vi "RobotSimulator.vi"() -> ()   [LabVIEW 2020]
uses:
  <vilib>/Utility/inputDevices.llb/joystickAcquire.vi
  <vilib>/Utility/inputDevices.llb/closeJoystick.vi
panel:
  out "?":dbl(knob) scale=-10.0..10.0
  out "Velocidade":dbl
  out "Trás Esq.":bool
  out "Frente Dir.":bool
  out "Trás Dir.":bool
  out "Frente Esq.":bool
  out "joystick info":T1(array[cluster])
  out "direction info":T2
  out "button info":T3
  out "axis info":T4
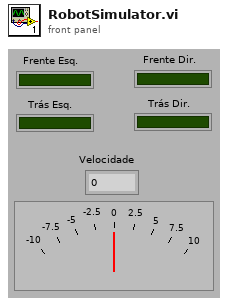
[diagram p1: front panel]
types:
  T1 = cluster{"axes total":u32, "buttons total":u32, "pov total":u32, "device name":string}[]
  T2 = cluster{"pov 1":i32, "pov 2":i32, "pov 3":i32, "pov 4":i32}
  T3 = cluster{"button 1":bool, "button 2":bool, "button 3":bool, "button 4":bool, "button 5":bool, "button 6":bool, "button 7":bool, "button 8":bool, "button 9":bool, "button 10":bool, "button 11":bool, "button 12":bool, "button 13":bool, "button 14":bool, "button 15":bool, "button 16":bool, "button 17":bool, "button 18":bool, "button 19":bool, "button 20":bool, "button 21":bool, "button 22":bool, "button 23":bool, "button 24":bool, "button 25":bool, "button 26":bool, "button 27":bool, "button 28":bool, "button 29":bool, "button 30":bool, "button 31":bool, "button 32":bool}
  T4 = cluster{"X axis":i32, "Y axis":i32, "Z axis":i32, "X axis rotation":i32, "Y axis rotation":i32, "Z axis rotation":i32, "U axis":i32, "V axis":i32}
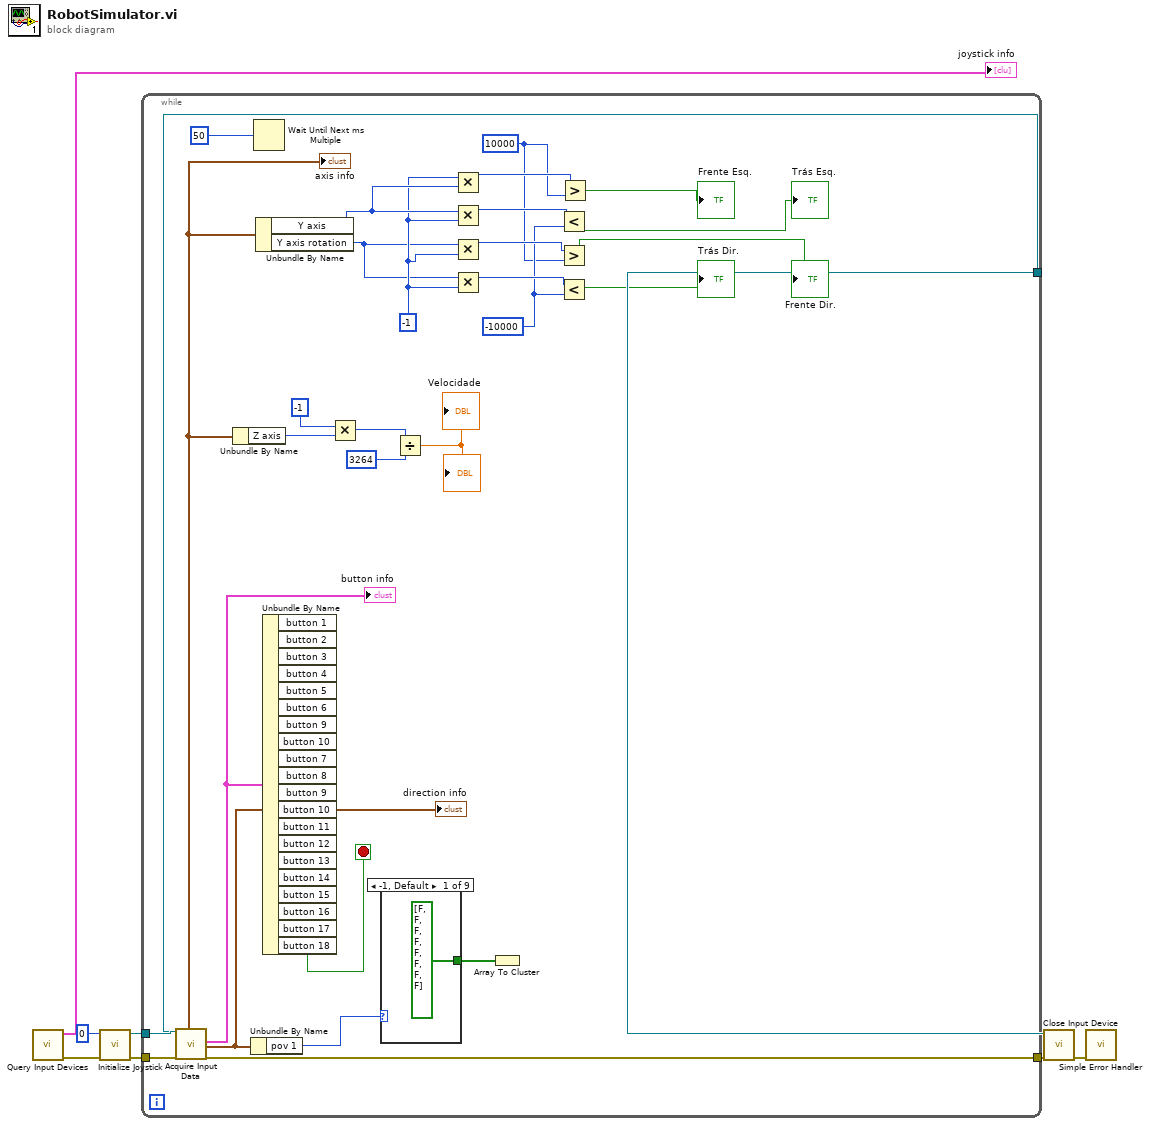
[diagram p0: block diagram]
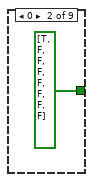
[diagram p2: hidden frame]
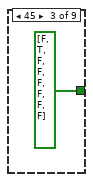
[diagram p3: hidden frame]
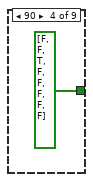
[diagram p4: hidden frame]
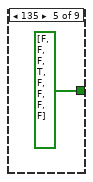
[diagram p5: hidden frame]
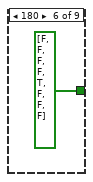
[diagram p6: hidden frame]
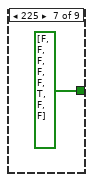
[diagram p7: hidden frame]
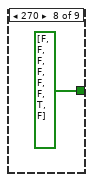
[diagram p8: hidden frame]
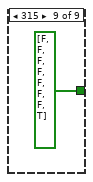
[diagram p9: hidden frame]
diagram:
  n1 = call <vilib>:"Query Input Devices.vi"() -> ("error out"=w2:errorcluster, "joystick info"=→"joystick info":T1)  [unwired: 1 in, 9 out]
  n2 = call <vilib>:"Initialize Joystick.vi"("error in (no error)"=w2, "device index"=0) -> ("error out"=w6:errorcluster, "device ID"=w7:refnum<k1>)  [unwired: 8 out]
  n3 = while {
    tunnel: w7 -> [w37]
    tunnel: w6 -> [w36]
    tunnel: [w35] -> w5
    tunnel: [w30] -> w4
    stop <- w29 stop-if-true
    w15 = 10000
    w16 = -10000
    w25 = -1
    n4 = call-poly <vilib>:"Acquire Input Data.vi"("device ID"=w37, "error in (no error)"=w36) -> ("device ID"=w35:refnum<k1>, "axis info"=w27:T4, "button info"=w34:T3, "direction info"=w33:T2, "error out"=w30:errorcluster)  [unwired: 13 out]
    "axis info" <- w27
    "button info" <- w34
    "direction info" <- w33
    n5 = Unbundle By Name(w27) -> ("Z axis"=w12:i32)
    n6 = Unbundle By Name(w33) -> ("pov 1"=w32:i32)
    n7 = Wait Until Next ms Multiple(millisecond multiple=u32 50) -> ()  [unwired: 1 out]
    n8 = Unbundle By Name(w27) -> ("Y axis"=w26:i32, "Y axis rotation"=w24:i32)
    n9 = Unbundle By Name(w34) -> ("button 7"=w29:bool)  [unwired: 19 out]
    n10 = Multiply(x=w12, y=-1) -> (x*y=w11:i32)
    n11 = case shown="-1, Default" w32 {
      tunnel: [bool[] [FALSE, FALSE, FALSE, FALSE, FALSE, FALSE, FALSE, FALSE] ("Array") bool[] [TRUE, FALSE, FALSE, FALSE, FALSE, FALSE, FALSE, FALSE] ("Array") bool[] [FALSE, TRUE, FALSE, FALSE, FALSE, FALSE, FALSE, FALSE] ("Array") bool[] [FALSE, FALSE, TRUE, FALSE, FALSE, FALSE, FALSE, FALSE] ("Array") bool[] [FALSE, FALSE, FALSE, TRUE, FALSE, FALSE, FALSE, FALSE] ("Array") bool[] [FALSE, FALSE, FALSE, FALSE, TRUE, FALSE, FALSE, FALSE] ("Array") bool[] [FALSE, FALSE, FALSE, FALSE, FALSE, TRUE, FALSE, FALSE] ("Array") bool[] [FALSE, FALSE, FALSE, FALSE, FALSE, FALSE, TRUE, FALSE] ("Array") bool[] [FALSE, FALSE, FALSE, FALSE, FALSE, FALSE, FALSE, TRUE] ("Array")] -> w31
      frame -1, Default {
      }
      frame 0 {
      }
      frame 45 {
      }
      frame 90 {
      }
      frame 135 {
      }
      frame 180 {
      }
      frame 225 {
      }
      frame 270 {
      }
      frame 315 {
      }
    }
    n12 = Divide(x=w11, y=3264) -> (x/y=→"Velocidade" →"?":dbl)
    n13 = Multiply(x=w25, y=w26) -> (x*y=w17:i32)
    n14 = Multiply(x=w26, y=w25) -> (x*y=w20:i32)
    n15 = Multiply(x=w24, y=w25) -> (x*y=w22:i32)
    n16 = Multiply(x=w24, y=w25) -> (x*y=w21:i32)
    n17 = Array To Cluster(array=w31) -> ()  [unwired: 1 out]
    n18 = Less?(x=w20, y=w16) -> (x < y?=→"Trás Esq.":bool)
    n19 = Greater?(x=w22, y=w15) -> (0:→"Frente Dir.":bool)
    n20 = Less?(x=w21, y=w16) -> (x < y?=→"Trás Dir.":bool)
    n21 = Greater?(x=w17, y=w15) -> (0:→"Frente Esq.":bool)
  }
  n22 = call-poly <vilib>:"Close Input Device.vi"("error in (no error)"=w4, "device ID"=w5) -> ("error out"=w1:errorcluster)  [unwired: 8 out]
  n23 = call <vilib>:"Simple Error Handler.vi"("error in (no error)"=w1) -> ()  [unwired: 1 in, 8 out]
